vi "Get Enq.vi"(8 "error in":errorcluster, 10 "Ident":string, 11 "Interactor in":refnum<class "Interactor.lvclass">) -> (0 "error out":errorcluster, 2 "Enq":refnum<class "Message Enqueuer.lvclass">, 3 "Interactor out":refnum<class "Interactor.lvclass">)   [LabVIEW 2024, in "Interactor.lvlib" / "Interactor.lvclass"]
uses:
  Interactor.lvclass
  <vilib>/ActorFramework/Message Enqueuer/Message Enqueuer.lvclass
  Interactor.lvclass/Interactor.ctl
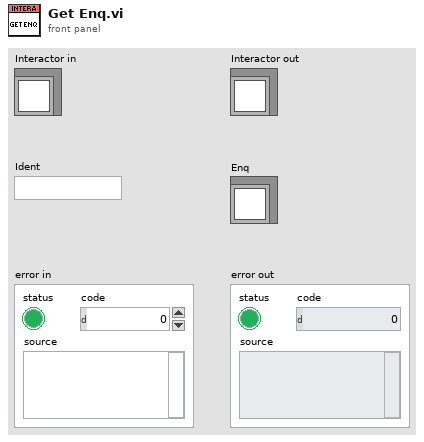
[diagram p1: front panel]
types:
  T1 = map{string, refnum<class "Message Enqueuer.lvclass">}
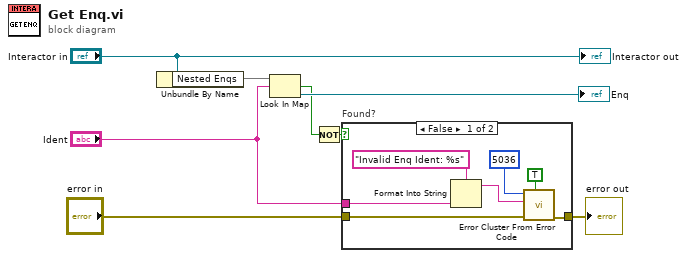
[diagram p0: block diagram]
diagram:
  n1 = Unbundle By Name("Interactor in") -> ("Nested Enqs"=w7:T1)
  n2 = Look In Map(map=w7, key="Ident") -> (key not found?=w5:bool, value=→"Enq":refnum<class "Message Enqueuer.lvclass">)  [unwired: 1 in]
  n3 = Not(x=w5) -> (.not. x?=w2:bool)
  n4 = case "Found?" shown="False" w2 {
    tunnel: [w15 w16] -> w4
    tunnel: "error in" -> [w14 w16]
    tunnel: "Ident" -> [w10 _]
    frame False {
      n5 = Format Into String(format string="Invalid Enq Ident: %s" ("error message (\"\")"), w10) -> (resulting string=w9:string)  [unwired: 2 in, 1 out]
      n6 = call <vilib>:"Error Cluster From Error Code.vi"("show call chain? (False)"=TRUE, "error in (no error)"=w14, "error message (\"\")"=w9, "error code (0)"=5036) -> ("error out"=w15:errorcluster)  [unwired: 5 in]
    }
    frame True {
    }
  }
  "error out" <- w4
  "Interactor out" <- "Interactor in"
